vi "S2C_OM8257_Proc_CacheState.vi"(7 "Label":string, 8 "Error In":errorcluster, 11 "Data In":string) -> (0 "Error Out":errorcluster, 3 "Data Out":string)   [LabVIEW 2015]
uses:
  S2C_OM8257_Proc_Globals.vi
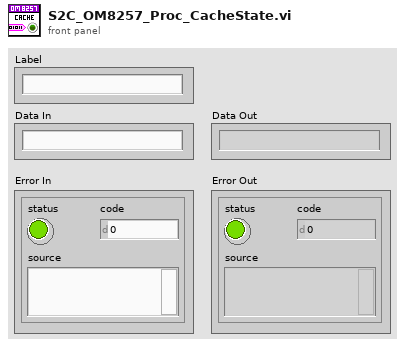
[diagram p1: front panel]
types:
  T1 = cluster{"Voltage (V)":u16, "High Limit Total (mA)":dbl, "Low Limit Total (mA)":dbl, "Ramp Up Time (s)":dbl, "Dwell Time (s)":dbl, "Arc Sense":u8, "Arc Detect":bool, "High Limit Real (mA)":dbl, "Low Limit Real (mA)":dbl, "Ramp Down Time (s)":dbl, "Continuity":bool, "Offset (mA)":dbl, "Auto Offset":bool, "DUT Output":bool, "Frequency (Hz)":u16, "Scanner?":bool, "Step Selection":i32, "Add Step":bool, "ACW-Scan":cluster{"Scan1":i32, "Scan2":i32, "Scan3":i32, "Scan4":i32, "Scan5":i32, "Scan6":i32, "Scan7":i32, "Scan8":i32, "Scan9":i32, "Scan10":i32, "Scan11":i32, "Scan12":i32, "Scan13":i32, "Scan14":i32, "Scan15":i32, "Scan16":i32}, "P1P1C1Exe":bool}
  T2 = cluster{"Voltage (V)":u16, "High Limit Total (mA)":dbl, "Low Limit Total (mA)":dbl, "Ramp Up Time (s)":dbl, "Dwell Time (s)":dbl, "Arc Sense":u8, "Arc Detect":bool, "High Limit Real (mA)":dbl, "Low Limit Real (mA)":dbl, "Ramp Down Time (s)":dbl, "Continuity":bool, "Offset (mA)":dbl, "Auto Offset":bool, "DUT Output":bool, "Frequency (Hz)":u16, "Scanner?":bool, "Step Selection":i32, "Add Step":bool, "Scan1":i32, "Scan2":i32, "Scan3":i32, "Scan4":i32, "Scan5":i32, "Scan6":i32, "Scan7":i32, "Scan8":i32, "Scan9":i32, "Scan10":i32, "Scan11":i32, "Scan12":i32, "Scan13":i32, "Scan14":i32, "Scan15":i32, "Scan16":i32}
  T3 = cluster{"Scan1":i32, "Scan2":i32, "Scan3":i32, "Scan4":i32, "Scan5":i32, "Scan6":i32, "Scan7":i32, "Scan8":i32, "Scan9":i32, "Scan10":i32, "Scan11":i32, "Scan12":i32, "Scan13":i32, "Scan14":i32, "Scan15":i32, "Scan16":i32}
  T4 = cluster{"Leakage-Hi (V)":dbl, "Leakage-Lo (V)":dbl, "Voltage-Hi (V)":dbl, "Voltage-Lo (V)":dbl, "Dwell (s)":dbl, "Delay (s)":dbl, "Offset (uA)":dbl, "AC Src Voltage (V)":dbl, "AC Src A-Hi (A)":dbl, "AC Source":bool, "AC Src Frequency":dbl, "Auto Offset":bool, "Reverse":bool, "Active Link":bool, "AC Src OC Fold":bool, "Neutral":bool, "Ground":bool, "Leakage":bool, "Ranging Mode":bool, "AC Src Output":bool, "AC Src Range":bool, "Measure Device":u16, "Probe":u16, "Filter Mode":u16, "Scanner?":bool, "Step Selection":i32, "Add Step":bool, "ACW-Scan":cluster{"Scan1":i32, "Scan2":i32, "Scan3":i32, "Scan4":i32, "Scan5":i32, "Scan6":i32, "Scan7":i32, "Scan8":i32, "Scan9":i32, "Scan10":i32, "Scan11":i32, "Scan12":i32, "Scan13":i32, "Scan14":i32, "Scan15":i32, "Scan16":i32}, "P1P2C1Exe":bool}
  T5 = cluster{"Leakage-Hi (V)":dbl, "Leakage-Lo (V)":dbl, "Voltage-Hi (V)":dbl, "Voltage-Lo (V)":dbl, "Dwell (s)":dbl, "Delay (s)":dbl, "Offset (uA)":dbl, "AC Src Voltage (V)":dbl, "AC Src A-Hi (A)":dbl, "AC Source":bool, "AC Src Frequency":dbl, "Auto Offset":bool, "Reverse":bool, "Active Link":bool, "AC Src OC Fold":bool, "Neutral":bool, "Ground":bool, "Leakage":bool, "Ranging Mode":bool, "AC Src Output":bool, "AC Src Range":bool, "Measure Device":u16, "Probe":u16, "Filter Mode":u16, "Scanner?":bool, "Step Selection":i32, "Add Step":bool, "Scan1":i32, "Scan2":i32, "Scan3":i32, "Scan4":i32, "Scan5":i32, "Scan6":i32, "Scan7":i32, "Scan8":i32, "Scan9":i32, "Scan10":i32, "Scan11":i32, "Scan12":i32, "Scan13":i32, "Scan14":i32, "Scan15":i32, "Scan16":i32}
  T6 = cluster{"Current (A)":dbl, "Voltage (V)":dbl, "Hi-Limit (mohm)":u16, "Lo-Limit (mhom)":u16, "Dwell (s)":dbl, "Offset (mhom)":u16, "Auto Offset":bool, "Frequency (Hz)":u16, "DualCHEK":u16, "Scanner Selection":i32, "Scanner?":bool, "Step Selection":i32, "Add Step":bool, "P1P3C1Exe":bool}
  T7 = cluster{"Current (A)":dbl, "Voltage (V)":dbl, "Hi-Limit (mohm)":u16, "Lo-Limit (mhom)":u16, "Dwell (s)":dbl, "Offset (mhom)":u16, "Auto Offset":bool, "Frequency (Hz)":u16, "DualCHEK":u16, "Scanner Selection":i32, "Scanner?":bool, "Step Selection":i32, "Add Step":bool}
  T8 = cluster{"Voltage-Hi (V)":dbl, "Voltage-Lo (V)":dbl, "Amp-Hi (A)":dbl, "Amp-Lo (A)":dbl, "Dwell (s)":dbl, "Delay (s)":dbl, "Leakage-Hi (mA)":dbl, "Leakage-Lo (mA)":dbl, "Power-Hi (W)":u16, "Power-Lo (W)":u16, "PF-Hi":dbl, "PF-Lo":dbl, "AC Src Voltage (V)":dbl, "AC Src A-Hi (A)":dbl, "AC Source":bool, "AC Src Frequency (Hz)":u16, "AC Src OC Fold":bool, "AC Src Output":bool, "AC Src Range":bool, "Active Link":bool, "Step Selection":i32, "Add Step":bool, "P1P4C1Exe":bool}
  T9 = cluster{"Voltage-Hi (V)":dbl, "Voltage-Lo (V)":dbl, "Amp-Hi (A)":dbl, "Amp-Lo (A)":dbl, "Dwell (s)":dbl, "Delay (s)":dbl, "Leakage-Hi (mA)":dbl, "Leakage-Lo (mA)":dbl, "Power-Hi (W)":u16, "Power-Lo (W)":u16, "PF-Lo":dbl, "PF-Hi":dbl, "AC Src Voltage (V)":dbl, "AC Src A-Hi (A)":dbl, "AC Source":bool, "AC Src Frequency (Hz)":u16, "AC Src OC Fold":bool, "AC Src Output":bool, "AC Src Range":bool, "Active Link":bool, "Step Selection":i32, "Add Step":bool}
  T10 = cluster{"Resource Name":refnum<visa-resource-name>, "Baud Rate":u32, "Data Bits":u16, "Parity":u16, "Stop Bits":u16, "Flow Control":u16, "Timeout":u32, "Reset":bool, "P1C1Exe":bool}
  T11 = cluster{"Resource Name":string, "Baud Rate":u32, "Data Bits":u16, "Parity":u16, "Stop Bits":u16, "Flow Control":u16, "Timeout":u32, "Reset":bool}
  T12 = cluster{"File Number":i32, "Filename":string, "P5C1Exe":bool}
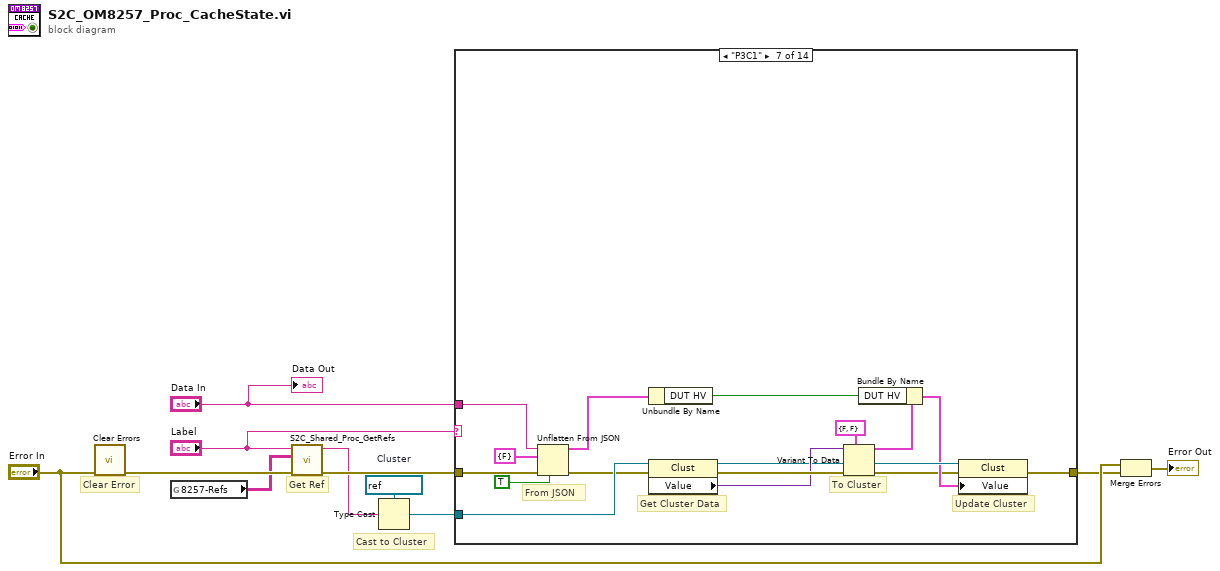
[diagram p0: block diagram]
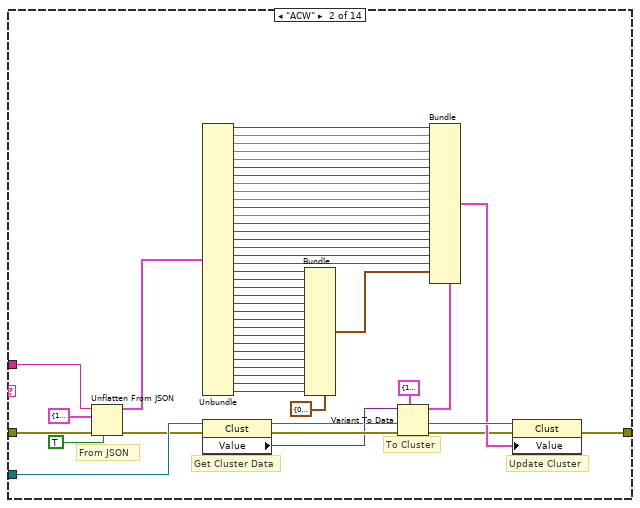
[diagram p3: hidden frame]
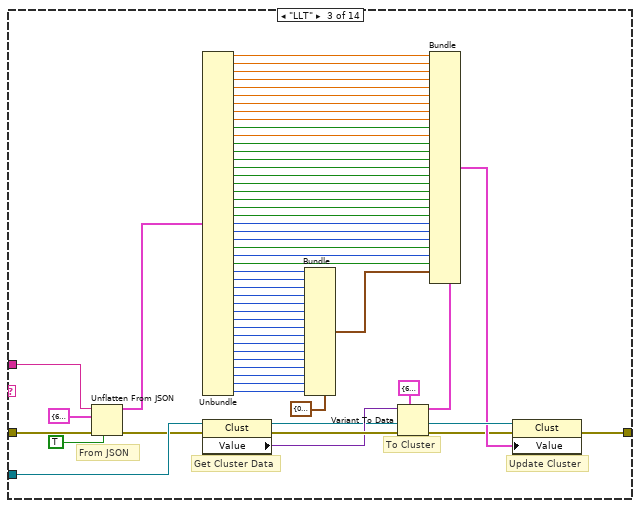
[diagram p4: hidden frame]
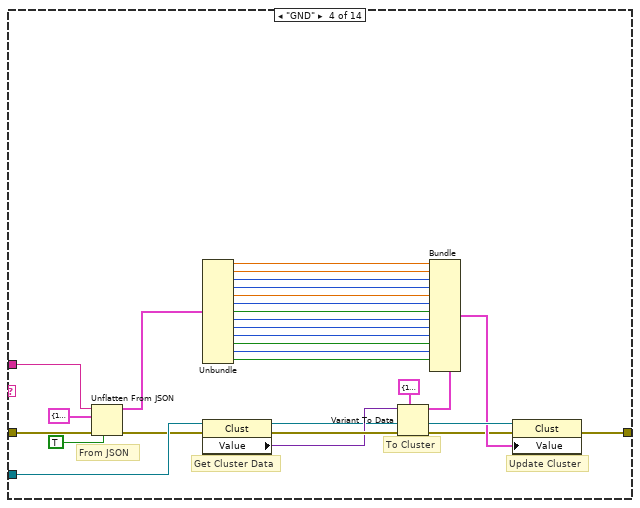
[diagram p5: hidden frame]
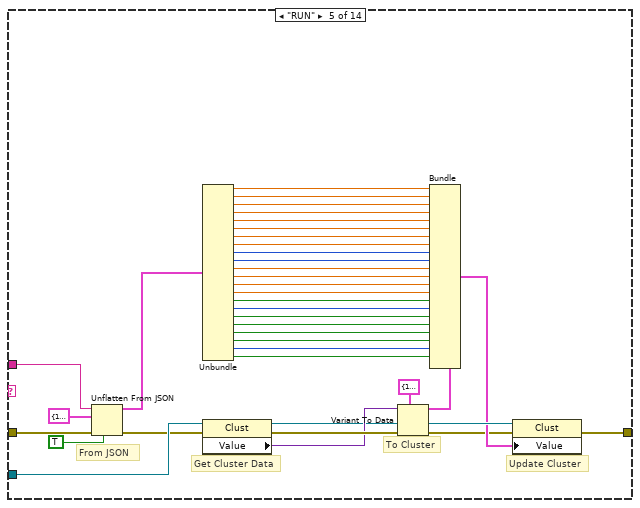
[diagram p6: hidden frame]
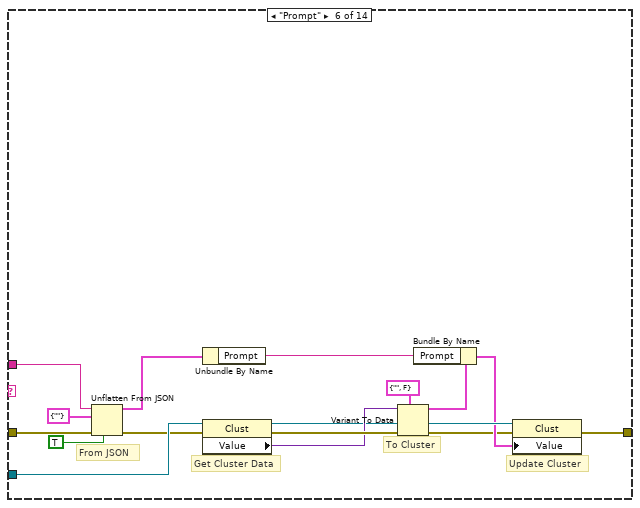
[diagram p7: hidden frame]
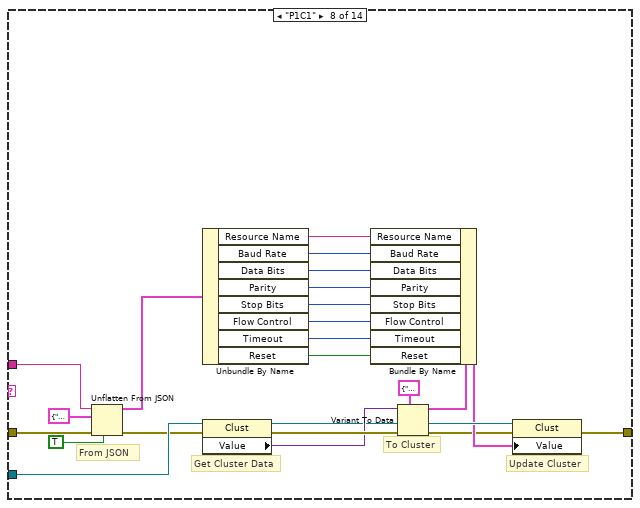
[diagram p8: hidden frame]
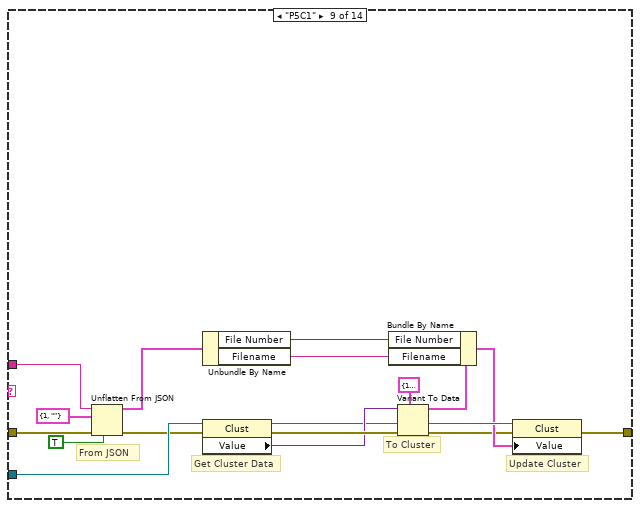
[diagram p9: hidden frame]
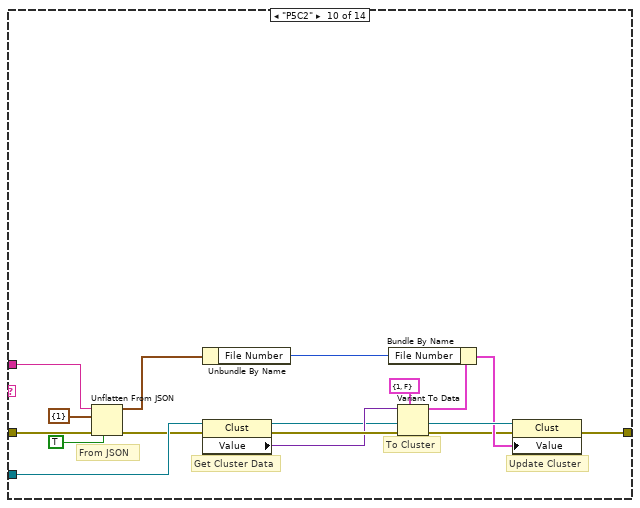
[diagram p10: hidden frame]
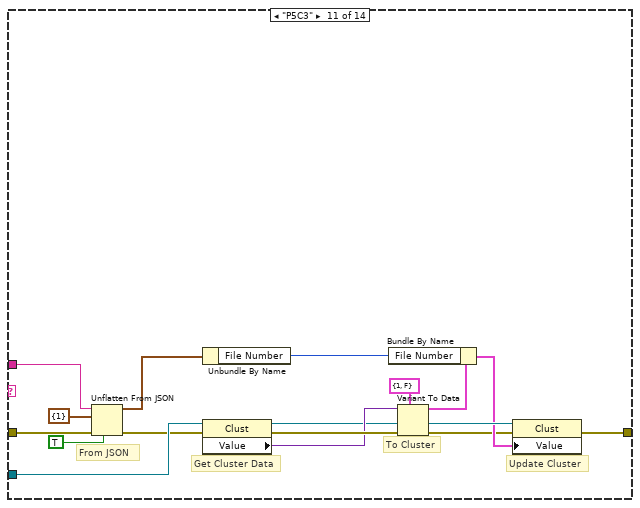
[diagram p11: hidden frame]
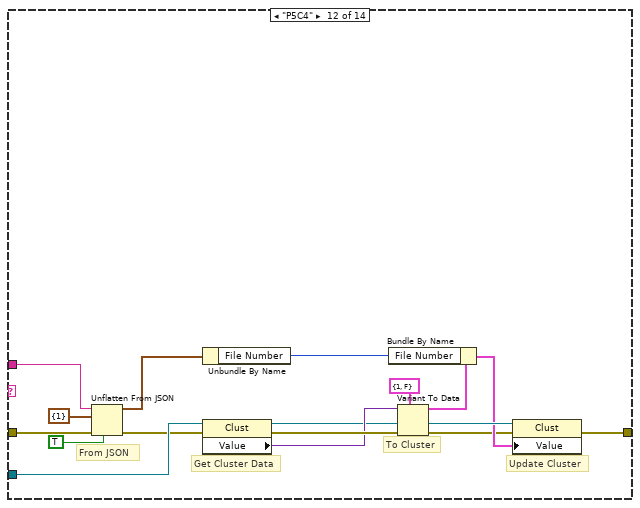
[diagram p12: hidden frame]
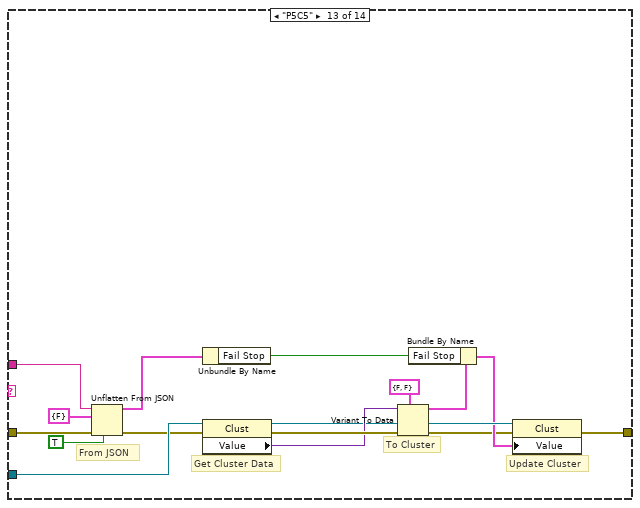
[diagram p13: hidden frame]
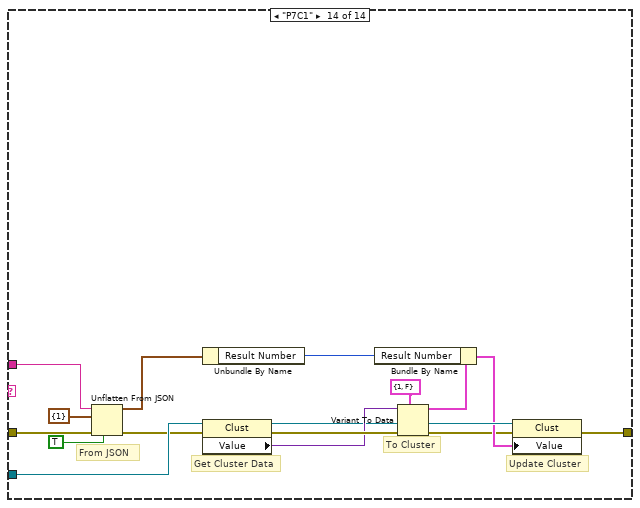
[diagram p14: hidden frame]
diagram:
  w7 = refnum<vi> refnum  # Cluster
  # "Cast to Cluster"
  # "Get Ref"
  # "Clear Error"
  n1 = call <vilib>:"Clear Errors.vi"("error in (no error)"="Error In") -> ("error out"=w4:errorcluster)  [unwired: 5 in, 1 out]
  n2 = global read "S2C_OM8257_Proc_Globals.vi" "8257-Refs"() -> (w1:string[][])
  n3 = call "S2C_Shared_Proc_GetRefs.vi"("Error In"=w4, "Refs"=w1, "Label"="Label") -> ("Error Out"=w9:errorcluster, "Reference"=w6:string)  [unwired: 7 in]
  n4 = Type Cast(type=w7, x=w6) -> (*(type *) &x=w5:refnum<vi>)
  n5 = case shown="\"P3C1\"" "Label" {
    tunnel: w9 -> [w12 w58 w118 w146 w183 w199 w215 w238 w255 w271 w287 w303 w319 w335]
    tunnel: [w12 w52 w112 w140 w177 w193 w209 w232 w249 w265 w281 w297 w313 w329] -> w2
    tunnel: w5 -> [_ w60 w120 w148 w185 w201 w217 w240 w257 w273 w289 w305 w321 w337]
    tunnel: "Data In" -> [_ w56 w116 w144 w181 w197 w213 w236 w253 w269 w285 w301 w317 w333]
    frame "Other", Default {
    }
    frame "ACW" {
      # "Update Cluster"
      # "To Cluster"
      # "Get Cluster Data"
      # "From JSON"
      n6 = Unflatten From JSON(JSON string=w56, type and defaults=T2 {"Voltage (V)"=1240, "High Limit Total (mA)"=10.0, "Low Limit Total (mA)"=0.0, "Ramp Up Time (s)"=0.1, "Dwell Time (s)"=1.0, "Arc Sense"=5, "Arc Detect"=FALSE, "High Limit Real (mA)"=10.0, "Low Limit Real (mA)"=0.0, "Ramp Down Time (s)"=0.0, "Continuity"=FALSE, "Offset (mA)"=0.0, "Auto Offset"=FALSE, "DUT Output"=FALSE, "Frequency (Hz)"=60, "Scanner?"=FALSE, "Step Selection"=1, "Add Step"=FALSE, "Scan1"=1, "Scan2"=1, "Scan3"=1, "Scan4"=1, "Scan5"=1, "Scan6"=1, "Scan7"=1, "Scan8"=1, "Scan9"=1, "Scan10"=1, "Scan11"=1, "Scan12"=1, "Scan13"=1, "Scan14"=1, "Scan15"=1, "Scan16"=1} ("ACW"), default null elements? (F)=TRUE, error in (no error)=w58) -> (value=w57:T2, error out=w55:errorcluster)  [unwired: 3 in]
      n7 = Unbundle(w57) -> ("Voltage (V)"=w50:u16, "High Limit Total (mA)"=w49:dbl, "Low Limit Total (mA)"=w48:dbl, "Ramp Up Time (s)"=w47:dbl, "Dwell Time (s)"=w46:dbl, "Arc Sense"=w45:u8, "Arc Detect"=w44:bool, "High Limit Real (mA)"=w43:dbl, "Low Limit Real (mA)"=w42:dbl, "Ramp Down Time (s)"=w41:dbl, "Continuity"=w40:bool, "Offset (mA)"=w39:dbl, "Auto Offset"=w38:bool, "DUT Output"=w37:bool, "Frequency (Hz)"=w36:u16, "Scanner?"=w35:bool, "Step Selection"=w34:i32, "Add Step"=w33:bool, "Scan1"=w31:i32, "Scan2"=w30:i32, "Scan3"=w29:i32, "Scan4"=w28:i32, "Scan5"=w27:i32, "Scan6"=w26:i32, "Scan7"=w25:i32, "Scan8"=w24:i32, "Scan9"=w23:i32, "Scan10"=w22:i32, "Scan11"=w21:i32, "Scan12"=w20:i32, "Scan13"=w19:i32, "Scan14"=w18:i32, "Scan15"=w17:i32, "Scan16"=w16:i32)
      n8 = property class="Clust"(reference=w60, error in=w55) -> (reference out=w54:refnum<vi>, error out=w63:errorcluster, "Value"=w62:variant)
      n9 = Bundle(cluster=T3 {"Scan1"=0, "Scan2"=0, "Scan3"=0, "Scan4"=0, "Scan5"=0, "Scan6"=0, "Scan7"=0, "Scan8"=0, "Scan9"=0, "Scan10"=0, "Scan11"=0, "Scan12"=0, "Scan13"=0, "Scan14"=0, "Scan15"=0, "Scan16"=0} ("ACW-Scan"), "Scan1"=w31, "Scan2"=w30, "Scan3"=w29, "Scan4"=w28, "Scan5"=w27, "Scan6"=w26, "Scan7"=w25, "Scan8"=w24, "Scan9"=w23, "Scan10"=w22, "Scan11"=w21, "Scan12"=w20, "Scan13"=w19, "Scan14"=w18, "Scan15"=w17, "Scan16"=w16) -> (w15:T3)
      n10 = Variant To Data(error in=w63, type=T1 {"Voltage (V)"=1240, "High Limit Total (mA)"=10.0, "Low Limit Total (mA)"=0.0, "Ramp Up Time (s)"=0.1, "Dwell Time (s)"=1.0, "Arc Sense"=5, "Arc Detect"=FALSE, "High Limit Real (mA)"=10.0, "Low Limit Real (mA)"=0.0, "Ramp Down Time (s)"=0.0, "Continuity"=FALSE, "Offset (mA)"=0.0, "Auto Offset"=FALSE, "DUT Output"=FALSE, "Frequency (Hz)"=60, "Scanner?"=FALSE, "Step Selection"=1, "Add Step"=FALSE, "ACW-Scan"={"Scan1"=1, "Scan2"=1, "Scan3"=1, "Scan4"=1, "Scan5"=1, "Scan6"=1, "Scan7"=1, "Scan8"=1, "Scan9"=1, "Scan10"=1, "Scan11"=1, "Scan12"=1, "Scan13"=1, "Scan14"=1, "Scan15"=1, "Scan16"=1}, "P1P1C1Exe"=FALSE} ("ACW"), Variant=w62) -> (data=w61:T1, error out=w51:errorcluster)
      n11 = Bundle(cluster=w61, "Voltage (V)"=w50, "High Limit Total (mA)"=w49, "Low Limit Total (mA)"=w48, "Ramp Up Time (s)"=w47, "Dwell Time (s)"=w46, "Arc Sense"=w45, "Arc Detect"=w44, "High Limit Real (mA)"=w43, "Low Limit Real (mA)"=w42, "Ramp Down Time (s)"=w41, "Continuity"=w40, "Offset (mA)"=w39, "Auto Offset"=w38, "DUT Output"=w37, "Frequency (Hz)"=w36, "Scanner?"=w35, "Step Selection"=w34, "Add Step"=w33, "ACW-Scan"=w15) -> (w53:T1)  [unwired: 1 in]
      n12 = property class="Clust"(reference=w54, error in=w51, "Value"=w53) -> (error out=w52:errorcluster)  [unwired: 1 out]
    }
    frame "LLT" {
      # "Update Cluster"
      # "To Cluster"
      # "Get Cluster Data"
      # "From JSON"
      n13 = Unflatten From JSON(JSON string=w116, type and defaults=T5 {"Leakage-Hi (V)"=6000.0, "Leakage-Lo (V)"=0.0, "Voltage-Hi (V)"=125.0, "Voltage-Lo (V)"=0.0, "Dwell (s)"=0.5, "Delay (s)"=1.0, "Offset (uA)"=10.0, "AC Src Voltage (V)"=115.0, "AC Src A-Hi (A)"=0.0, "AC Source"=FALSE, "AC Src Frequency"=60.0, "Auto Offset"=FALSE, "Reverse"=FALSE, "Active Link"=FALSE, "AC Src OC Fold"=FALSE, "Neutral"=FALSE, "Ground"=FALSE, "Leakage"=FALSE, "Ranging Mode"=FALSE, "AC Src Output"=TRUE, "AC Src Range"=TRUE, "Measure Device"=0, "Probe"=0, "Filter Mode"=0, "Scanner?"=FALSE, "Step Selection"=1, "Add Step"=FALSE, "Scan1"=1, "Scan2"=1, "Scan3"=1, "Scan4"=1, "Scan5"=1, "Scan6"=1, "Scan7"=1, "Scan8"=1, "Scan9"=1, "Scan10"=1, "Scan11"=1, "Scan12"=1, "Scan13"=1, "Scan14"=1, "Scan15"=1, "Scan16"=1} ("LLT"), default null elements? (F)=TRUE, error in (no error)=w118) -> (value=w117:T5, error out=w115:errorcluster)  [unwired: 3 in]
      n14 = Unbundle(w117) -> ("Leakage-Hi (V)"=w90:dbl, "Leakage-Lo (V)"=w89:dbl, "Voltage-Hi (V)"=w88:dbl, "Voltage-Lo (V)"=w87:dbl, "Dwell (s)"=w86:dbl, "Delay (s)"=w85:dbl, "Offset (uA)"=w84:dbl, "AC Src Voltage (V)"=w83:dbl, "AC Src A-Hi (A)"=w82:dbl, "AC Source"=w81:bool, "AC Src Frequency"=w80:dbl, "Auto Offset"=w79:bool, "Reverse"=w78:bool, "Active Link"=w77:bool, "AC Src OC Fold"=w76:bool, "Neutral"=w75:bool, "Ground"=w74:bool, "Leakage"=w73:bool, "Ranging Mode"=w72:bool, "AC Src Output"=w71:bool, "AC Src Range"=w70:bool, "Measure Device"=w69:u16, "Probe"=w68:u16, "Filter Mode"=w67:u16, "Scanner?"=w66:bool, "Step Selection"=w65:i32, "Add Step"=w64:bool, "Scan1"=w109:i32, "Scan2"=w108:i32, "Scan3"=w107:i32, "Scan4"=w106:i32, "Scan5"=w105:i32, "Scan6"=w104:i32, "Scan7"=w103:i32, "Scan8"=w102:i32, "Scan9"=w101:i32, "Scan10"=w100:i32, "Scan11"=w99:i32, "Scan12"=w98:i32, "Scan13"=w97:i32, "Scan14"=w96:i32, "Scan15"=w95:i32, "Scan16"=w94:i32)
      n15 = property class="Clust"(reference=w120, error in=w115) -> (reference out=w114:refnum<vi>, error out=w123:errorcluster, "Value"=w122:variant)
      n16 = Bundle(cluster=T3 {"Scan1"=0, "Scan2"=0, "Scan3"=0, "Scan4"=0, "Scan5"=0, "Scan6"=0, "Scan7"=0, "Scan8"=0, "Scan9"=0, "Scan10"=0, "Scan11"=0, "Scan12"=0, "Scan13"=0, "Scan14"=0, "Scan15"=0, "Scan16"=0} ("ACW-Scan"), "Scan1"=w109, "Scan2"=w108, "Scan3"=w107, "Scan4"=w106, "Scan5"=w105, "Scan6"=w104, "Scan7"=w103, "Scan8"=w102, "Scan9"=w101, "Scan10"=w100, "Scan11"=w99, "Scan12"=w98, "Scan13"=w97, "Scan14"=w96, "Scan15"=w95, "Scan16"=w94) -> (w93:T3)
      n17 = Variant To Data(error in=w123, type=T4 {"Leakage-Hi (V)"=6000.0, "Leakage-Lo (V)"=0.0, "Voltage-Hi (V)"=125.0, "Voltage-Lo (V)"=0.0, "Dwell (s)"=0.5, "Delay (s)"=1.0, "Offset (uA)"=10.0, "AC Src Voltage (V)"=115.0, "AC Src A-Hi (A)"=0.0, "AC Source"=FALSE, "AC Src Frequency"=60.0, "Auto Offset"=FALSE, "Reverse"=FALSE, "Active Link"=FALSE, "AC Src OC Fold"=FALSE, "Neutral"=FALSE, "Ground"=FALSE, "Leakage"=FALSE, "Ranging Mode"=FALSE, "AC Src Output"=TRUE, "AC Src Range"=TRUE, "Measure Device"=0, "Probe"=0, "Filter Mode"=0, "Scanner?"=FALSE, "Step Selection"=1, "Add Step"=FALSE, "ACW-Scan"={"Scan1"=1, "Scan2"=1, "Scan3"=1, "Scan4"=1, "Scan5"=1, "Scan6"=1, "Scan7"=1, "Scan8"=1, "Scan9"=1, "Scan10"=1, "Scan11"=1, "Scan12"=1, "Scan13"=1, "Scan14"=1, "Scan15"=1, "Scan16"=1}, "P1P2C1Exe"=FALSE} ("LLT"), Variant=w122) -> (data=w121:T4, error out=w111:errorcluster)
      n18 = Bundle(cluster=w121, "Leakage-Hi (V)"=w90, "Leakage-Lo (V)"=w89, "Voltage-Hi (V)"=w88, "Voltage-Lo (V)"=w87, "Dwell (s)"=w86, "Delay (s)"=w85, "Offset (uA)"=w84, "AC Src Voltage (V)"=w83, "AC Src A-Hi (A)"=w82, "AC Source"=w81, "AC Src Frequency"=w80, "Auto Offset"=w79, "Reverse"=w78, "Active Link"=w77, "AC Src OC Fold"=w76, "Neutral"=w75, "Ground"=w74, "Leakage"=w73, "Ranging Mode"=w72, "AC Src Output"=w71, "AC Src Range"=w70, "Measure Device"=w69, "Probe"=w68, "Filter Mode"=w67, "Scanner?"=w66, "Step Selection"=w65, "Add Step"=w64, "ACW-Scan"=w93) -> (w113:T4)  [unwired: 1 in]
      n19 = property class="Clust"(reference=w114, error in=w111, "Value"=w113) -> (error out=w112:errorcluster)  [unwired: 1 out]
    }
    frame "GND" {
      # "Update Cluster"
      # "To Cluster"
      # "Get Cluster Data"
      # "From JSON"
      n20 = Unflatten From JSON(JSON string=w144, type and defaults=T7 {"Current (A)"=1240.0, "Voltage (V)"=10.0, "Hi-Limit (mohm)"=100, "Lo-Limit (mhom)"=0, "Dwell (s)"=1.0, "Offset (mhom)"=0, "Auto Offset"=FALSE, "Frequency (Hz)"=60, "DualCHEK"=0, "Scanner Selection"=0, "Scanner?"=FALSE, "Step Selection"=1, "Add Step"=FALSE} ("GND"), default null elements? (F)=TRUE, error in (no error)=w146) -> (value=w145:T7, error out=w143:errorcluster)  [unwired: 3 in]
      n21 = Unbundle(w145) -> ("Current (A)"=w138:dbl, "Voltage (V)"=w137:dbl, "Hi-Limit (mohm)"=w136:u16, "Lo-Limit (mhom)"=w135:u16, "Dwell (s)"=w134:dbl, "Offset (mhom)"=w133:u16, "Auto Offset"=w127:bool, "Frequency (Hz)"=w132:u16, "DualCHEK"=w131:u16, "Scanner Selection"=w126:i32, "Scanner?"=w125:bool, "Step Selection"=w124:i32, "Add Step"=w130:bool)
      n22 = property class="Clust"(reference=w148, error in=w143) -> (reference out=w142:refnum<vi>, error out=w151:errorcluster, "Value"=w150:variant)
      n23 = Variant To Data(error in=w151, type=T6 {"Current (A)"=1240.0, "Voltage (V)"=10.0, "Hi-Limit (mohm)"=100, "Lo-Limit (mhom)"=0, "Dwell (s)"=1.0, "Offset (mhom)"=0, "Auto Offset"=FALSE, "Frequency (Hz)"=60, "DualCHEK"=0, "Scanner Selection"=0, "Scanner?"=FALSE, "Step Selection"=1, "Add Step"=FALSE, "P1P3C1Exe"=FALSE} ("GND"), Variant=w150) -> (data=w149:T6, error out=w139:errorcluster)
      n24 = Bundle(cluster=w149, "Current (A)"=w138, "Voltage (V)"=w137, "Hi-Limit (mohm)"=w136, "Lo-Limit (mhom)"=w135, "Dwell (s)"=w134, "Offset (mhom)"=w133, "Auto Offset"=w127, "Frequency (Hz)"=w132, "DualCHEK"=w131, "Scanner Selection"=w126, "Scanner?"=w125, "Step Selection"=w124, "Add Step"=w130) -> (w141:T6)  [unwired: 1 in]
      n25 = property class="Clust"(reference=w142, error in=w139, "Value"=w141) -> (error out=w140:errorcluster)  [unwired: 1 out]
    }
    frame "RUN" {
      # "Update Cluster"
      # "To Cluster"
      # "Get Cluster Data"
      # "From JSON"
      n26 = Unflatten From JSON(JSON string=w181, type and defaults=T9 {"Voltage-Hi (V)"=125.0, "Voltage-Lo (V)"=0.0, "Amp-Hi (A)"=10.0, "Amp-Lo (A)"=0.0, "Dwell (s)"=1.0, "Delay (s)"=0.2, "Leakage-Hi (mA)"=10.0, "Leakage-Lo (mA)"=0.0, "Power-Hi (W)"=1000, "Power-Lo (W)"=0, "PF-Lo"=0.0, "PF-Hi"=1.0, "AC Src Voltage (V)"=115.0, "AC Src A-Hi (A)"=0.0, "AC Source"=FALSE, "AC Src Frequency (Hz)"=60, "AC Src OC Fold"=FALSE, "AC Src Output"=TRUE, "AC Src Range"=TRUE, "Active Link"=FALSE, "Step Selection"=1, "Add Step"=FALSE} ("RUN"), default null elements? (F)=TRUE, error in (no error)=w183) -> (value=w182:T9, error out=w180:errorcluster)  [unwired: 3 in]
      n27 = Unbundle(w182) -> ("Voltage-Hi (V)"=w175:dbl, "Voltage-Lo (V)"=w174:dbl, "Amp-Hi (A)"=w173:dbl, "Amp-Lo (A)"=w172:dbl, "Dwell (s)"=w171:dbl, "Delay (s)"=w170:dbl, "Leakage-Hi (mA)"=w166:dbl, "Leakage-Lo (mA)"=w169:dbl, "Power-Hi (W)"=w168:u16, "Power-Lo (W)"=w165:u16, "PF-Lo"=w164:dbl, "PF-Hi"=w163:dbl, "AC Src Voltage (V)"=w167:dbl, "AC Src A-Hi (A)"=w160:dbl, "AC Source"=w159:bool, "AC Src Frequency (Hz)"=w158:u16, "AC Src OC Fold"=w157:bool, "AC Src Output"=w156:bool, "AC Src Range"=w155:bool, "Active Link"=w154:bool, "Step Selection"=w153:i32, "Add Step"=w152:bool)
      n28 = property class="Clust"(reference=w185, error in=w180) -> (reference out=w179:refnum<vi>, error out=w188:errorcluster, "Value"=w187:variant)
      n29 = Variant To Data(error in=w188, type=T8 {"Voltage-Hi (V)"=125.0, "Voltage-Lo (V)"=0.0, "Amp-Hi (A)"=10.0, "Amp-Lo (A)"=0.0, "Dwell (s)"=1.0, "Delay (s)"=0.2, "Leakage-Hi (mA)"=10.0, "Leakage-Lo (mA)"=0.0, "Power-Hi (W)"=1000, "Power-Lo (W)"=0, "PF-Hi"=1.0, "PF-Lo"=0.0, "AC Src Voltage (V)"=115.0, "AC Src A-Hi (A)"=0.0, "AC Source"=FALSE, "AC Src Frequency (Hz)"=60, "AC Src OC Fold"=FALSE, "AC Src Output"=TRUE, "AC Src Range"=TRUE, "Active Link"=FALSE, "Step Selection"=1, "Add Step"=FALSE, "P1P4C1Exe"=FALSE} ("RUN"), Variant=w187) -> (data=w186:T8, error out=w176:errorcluster)
      n30 = Bundle(cluster=w186, "Voltage-Hi (V)"=w175, "Voltage-Lo (V)"=w174, "Amp-Hi (A)"=w173, "Amp-Lo (A)"=w172, "Dwell (s)"=w171, "Delay (s)"=w170, "Leakage-Hi (mA)"=w166, "Leakage-Lo (mA)"=w169, "Power-Hi (W)"=w168, "Power-Lo (W)"=w165, "PF-Hi"=w164, "PF-Lo"=w163, "AC Src Voltage (V)"=w167, "AC Src A-Hi (A)"=w160, "AC Source"=w159, "AC Src Frequency (Hz)"=w158, "AC Src OC Fold"=w157, "AC Src Output"=w156, "AC Src Range"=w155, "Active Link"=w154, "Step Selection"=w153, "Add Step"=w152) -> (w178:T8)  [unwired: 1 in]
      n31 = property class="Clust"(reference=w179, error in=w176, "Value"=w178) -> (error out=w177:errorcluster)  [unwired: 1 out]
    }
    frame "Prompt" {
      # "Update Cluster"
      # "To Cluster"
      # "Get Cluster Data"
      # "From JSON"
      n32 = Unflatten From JSON(JSON string=w197, type and defaults=cluster{"Prompt":string} {"Prompt"=""} ("Prompt"), default null elements? (F)=TRUE, error in (no error)=w199) -> (value=w198:cluster{"Prompt":string}, error out=w196:errorcluster)  [unwired: 3 in]
      n33 = Unbundle By Name(w198) -> ("Prompt"=w190:string)
      n34 = property class="Clust"(reference=w201, error in=w196) -> (reference out=w195:refnum<vi>, error out=w204:errorcluster, "Value"=w203:variant)
      n35 = Variant To Data(error in=w204, type=cluster{"Prompt":string, "P1P5C1Exe":bool} {"Prompt"="", "P1P5C1Exe"=FALSE} ("Prompt"), Variant=w203) -> (data=w202:cluster{"Prompt":string, "P1P5C1Exe":bool}, error out=w192:errorcluster)
      n36 = Bundle By Name(cluster=w202, "Prompt"=w190) -> (w194:cluster{"Prompt":string, "P1P5C1Exe":bool})
      n37 = property class="Clust"(reference=w195, error in=w192, "Value"=w194) -> (error out=w193:errorcluster)  [unwired: 1 out]
    }
    frame "P3C1" {
      # "Update Cluster"
      # "To Cluster"
      # "Get Cluster Data"
      # "From JSON"
      n38 = Unflatten From JSON(JSON string=w213, type and defaults=cluster{"DUT HV":bool} {"DUT HV"=FALSE} ("P3C1"), default null elements? (F)=TRUE, error in (no error)=w215) -> (value=w214:cluster{"DUT HV":bool}, error out=w212:errorcluster)  [unwired: 3 in]
      n39 = Unbundle By Name(w214) -> ("DUT HV"=w207:bool)
      n40 = property class="Clust"(reference=w217, error in=w212) -> (reference out=w211:refnum<vi>, error out=w220:errorcluster, "Value"=w219:variant)
      n41 = Variant To Data(error in=w220, type=cluster{"DUT HV":bool, "P3C1Exe":bool} {"DUT HV"=FALSE, "P3C1Exe"=FALSE} ("P3C1"), Variant=w219) -> (data=w218:cluster{"DUT HV":bool, "P3C1Exe":bool}, error out=w208:errorcluster)
      n42 = Bundle By Name(cluster=w218, "DUT HV"=w207) -> (w210:cluster{"DUT HV":bool, "P3C1Exe":bool})
      n43 = property class="Clust"(reference=w211, error in=w208, "Value"=w210) -> (error out=w209:errorcluster)  [unwired: 1 out]
    }
    frame "P1C1" {
      # "Update Cluster"
      # "To Cluster"
      # "Get Cluster Data"
      # "From JSON"
      n44 = Unflatten From JSON(JSON string=w236, type and defaults=T11 {"Resource Name"="", "Baud Rate"=0, "Data Bits"=0, "Parity"=0, "Stop Bits"=10, "Flow Control"=0, "Timeout"=0, "Reset"=FALSE} ("P1C1"), default null elements? (F)=TRUE, error in (no error)=w238) -> (value=w237:T11, error out=w235:errorcluster)  [unwired: 3 in]
      n45 = Unbundle By Name(w237) -> ("Resource Name"=w228:string, "Baud Rate"=w227:u32, "Data Bits"=w226:u16, "Parity"=w225:u16, "Stop Bits"=w224:u16, "Flow Control"=w223:u16, "Timeout"=w222:u32, "Reset"=w221:bool)
      n46 = property class="Clust"(reference=w240, error in=w235) -> (reference out=w234:refnum<vi>, error out=w243:errorcluster, "Value"=w242:variant)
      n47 = Variant To Data(error in=w243, type=T10 {"Resource Name"="", "Baud Rate"=0, "Data Bits"=7, "Parity"=2, "Stop Bits"=15, "Flow Control"=3, "Timeout"=0, "Reset"=FALSE, "P1C1Exe"=FALSE} ("P1C1"), Variant=w242) -> (data=w241:T10, error out=w231:errorcluster)
      n48 = Bundle By Name(cluster=w241, "Resource Name"=w228, "Baud Rate"=w227, "Data Bits"=w226, "Parity"=w225, "Stop Bits"=w224, "Flow Control"=w223, "Timeout"=w222, "Reset"=w221) -> (w233:T10)
      n49 = property class="Clust"(reference=w234, error in=w231, "Value"=w233) -> (error out=w232:errorcluster)  [unwired: 1 out]
    }
    frame "P5C1" {
      # "Update Cluster"
      # "To Cluster"
      # "Get Cluster Data"
      # "From JSON"
      n50 = Unflatten From JSON(JSON string=w253, type and defaults=cluster{"File Number":i32, "Filename":string} {"File Number"=1, "Filename"=""} ("P5C1"), default null elements? (F)=TRUE, error in (no error)=w255) -> (value=w254:cluster{"File Number":i32, "Filename":string}, error out=w252:errorcluster)  [unwired: 3 in]
      n51 = Unbundle By Name(w254) -> ("File Number"=w247:i32, "Filename"=w244:string)
      n52 = property class="Clust"(reference=w257, error in=w252) -> (reference out=w251:refnum<vi>, error out=w260:errorcluster, "Value"=w259:variant)
      n53 = Variant To Data(error in=w260, type=T12 {"File Number"=1, "Filename"="", "P5C1Exe"=FALSE} ("P5C1"), Variant=w259) -> (data=w258:T12, error out=w248:errorcluster)
      n54 = Bundle By Name(cluster=w258, "File Number"=w247, "Filename"=w244) -> (w250:T12)
      n55 = property class="Clust"(reference=w251, error in=w248, "Value"=w250) -> (error out=w249:errorcluster)  [unwired: 1 out]
    }
    frame "P5C2" {
      # "Update Cluster"
      # "To Cluster"
      # "Get Cluster Data"
      # "From JSON"
      n56 = Unflatten From JSON(JSON string=w269, type and defaults=cluster{"File Number":u16} {"File Number"=1} ("P5C2"), default null elements? (F)=TRUE, error in (no error)=w271) -> (value=w270:cluster{"File Number":u16}, error out=w268:errorcluster)  [unwired: 3 in]
      n57 = Unbundle By Name(w270) -> ("File Number"=w263:u16)
      n58 = property class="Clust"(reference=w273, error in=w268) -> (reference out=w267:refnum<vi>, error out=w276:errorcluster, "Value"=w275:variant)
      n59 = Variant To Data(error in=w276, type=cluster{"File Number":u16, "P5C2Exe":bool} {"File Number"=1, "P5C2Exe"=FALSE} ("P5C2"), Variant=w275) -> (data=w274:cluster{"File Number":u16, "P5C2Exe":bool}, error out=w264:errorcluster)
      n60 = Bundle By Name(cluster=w274, "File Number"=w263) -> (w266:cluster{"File Number":u16, "P5C2Exe":bool})
      n61 = property class="Clust"(reference=w267, error in=w264, "Value"=w266) -> (error out=w265:errorcluster)  [unwired: 1 out]
    }
    frame "P5C3" {
      # "Update Cluster"
      # "To Cluster"
      # "Get Cluster Data"
      # "From JSON"
      n62 = Unflatten From JSON(JSON string=w285, type and defaults=cluster{"File Number":u16} {"File Number"=1} ("P5C2"), default null elements? (F)=TRUE, error in (no error)=w287) -> (value=w286:cluster{"File Number":u16}, error out=w284:errorcluster)  [unwired: 3 in]
      n63 = Unbundle By Name(w286) -> ("File Number"=w279:u16)
      n64 = property class="Clust"(reference=w289, error in=w284) -> (reference out=w283:refnum<vi>, error out=w292:errorcluster, "Value"=w291:variant)
      n65 = Variant To Data(error in=w292, type=cluster{"File Number":u16, "P5C2Exe":bool} {"File Number"=1, "P5C2Exe"=FALSE} ("P5C2"), Variant=w291) -> (data=w290:cluster{"File Number":u16, "P5C2Exe":bool}, error out=w280:errorcluster)
      n66 = Bundle By Name(cluster=w290, "File Number"=w279) -> (w282:cluster{"File Number":u16, "P5C2Exe":bool})
      n67 = property class="Clust"(reference=w283, error in=w280, "Value"=w282) -> (error out=w281:errorcluster)  [unwired: 1 out]
    }
    frame "P5C4" {
      # "Update Cluster"
      # "To Cluster"
      # "Get Cluster Data"
      # "From JSON"
      n68 = Unflatten From JSON(JSON string=w301, type and defaults=cluster{"File Number":u16} {"File Number"=1} ("P5C2"), default null elements? (F)=TRUE, error in (no error)=w303) -> (value=w302:cluster{"File Number":u16}, error out=w300:errorcluster)  [unwired: 3 in]
      n69 = Unbundle By Name(w302) -> ("File Number"=w295:u16)
      n70 = property class="Clust"(reference=w305, error in=w300) -> (reference out=w299:refnum<vi>, error out=w308:errorcluster, "Value"=w307:variant)
      n71 = Variant To Data(error in=w308, type=cluster{"File Number":u16, "P5C2Exe":bool} {"File Number"=1, "P5C2Exe"=FALSE} ("P5C2"), Variant=w307) -> (data=w306:cluster{"File Number":u16, "P5C2Exe":bool}, error out=w296:errorcluster)
      n72 = Bundle By Name(cluster=w306, "File Number"=w295) -> (w298:cluster{"File Number":u16, "P5C2Exe":bool})
      n73 = property class="Clust"(reference=w299, error in=w296, "Value"=w298) -> (error out=w297:errorcluster)  [unwired: 1 out]
    }
    frame "P5C5" {
      # "Update Cluster"
      # "To Cluster"
      # "Get Cluster Data"
      # "From JSON"
      n74 = Unflatten From JSON(JSON string=w317, type and defaults=cluster{"Fail Stop":bool} {"Fail Stop"=FALSE} ("P5C5"), default null elements? (F)=TRUE, error in (no error)=w319) -> (value=w318:cluster{"Fail Stop":bool}, error out=w316:errorcluster)  [unwired: 3 in]
      n75 = Unbundle By Name(w318) -> ("Fail Stop"=w311:bool)
      n76 = property class="Clust"(reference=w321, error in=w316) -> (reference out=w315:refnum<vi>, error out=w324:errorcluster, "Value"=w323:variant)
      n77 = Variant To Data(error in=w324, type=cluster{"Fail Stop":bool, "P5C5Exe":bool} {"Fail Stop"=FALSE, "P5C5Exe"=FALSE} ("P5C5"), Variant=w323) -> (data=w322:cluster{"Fail Stop":bool, "P5C5Exe":bool}, error out=w312:errorcluster)
      n78 = Bundle By Name(cluster=w322, "Fail Stop"=w311) -> (w314:cluster{"Fail Stop":bool, "P5C5Exe":bool})
      n79 = property class="Clust"(reference=w315, error in=w312, "Value"=w314) -> (error out=w313:errorcluster)  [unwired: 1 out]
    }
    frame "P7C1" {
      # "Update Cluster"
      # "To Cluster"
      # "Get Cluster Data"
      # "From JSON"
      n80 = Unflatten From JSON(JSON string=w333, type and defaults=cluster{"Result Number":i32} {"Result Number"=1} ("P7C1"), default null elements? (F)=TRUE, error in (no error)=w335) -> (value=w334:cluster{"Result Number":i32}, error out=w332:errorcluster)  [unwired: 3 in]
      n81 = Unbundle By Name(w334) -> ("Result Number"=w327:i32)
      n82 = property class="Clust"(reference=w337, error in=w332) -> (reference out=w331:refnum<vi>, error out=w340:errorcluster, "Value"=w339:variant)
      n83 = Variant To Data(error in=w340, type=cluster{"Result Number":i32, "P7C1Exe":bool} {"Result Number"=1, "P7C1Exe"=FALSE} ("P7C1"), Variant=w339) -> (data=w338:cluster{"Result Number":i32, "P7C1Exe":bool}, error out=w328:errorcluster)
      n84 = Bundle By Name(cluster=w338, "Result Number"=w327) -> (w330:cluster{"Result Number":i32, "P7C1Exe":bool})
      n85 = property class="Clust"(reference=w331, error in=w328, "Value"=w330) -> (error out=w329:errorcluster)  [unwired: 1 out]
    }
  }
  n86 = Merge Errors("Error In", w2) -> (→"Error Out":errorcluster)
  "Data Out" <- "Data In"
